vi "Constants.vi"() -> (14 "MetersInPixel":dbl, 15 "RobotLength(Px)":i16, 16 "RobotWidth(Px)":i16, 17 "PictureCenterPoint":cluster{"x":i16, "y":i16}={"x"=250, "y"=250})   [LabVIEW 2009, in "Host.lvlib" / "Draw.lvlib"]
uses:
  Draw.lvlib
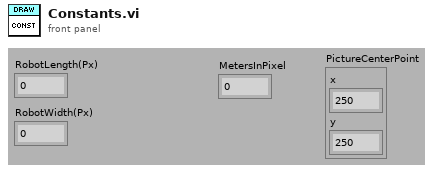
[diagram p1: front panel]
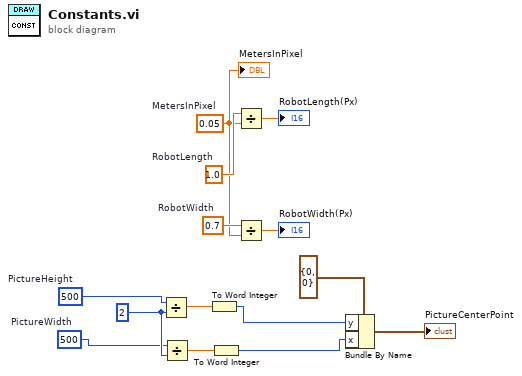
[diagram p0: block diagram]
diagram:
  w8 = i16 2 ("y")
  w7 = i16 500  # PictureWidth
  w9 = i16 500  # PictureHeight
  w12 = 0.7  # RobotWidth
  w14 = 1.0  # RobotLength
  w11 = 0.05  # MetersInPixel
  n1 = Divide(x=w9, y=w8) -> (x/y=w6:dbl)
  n2 = Divide(x=w7, y=w8) -> (x/y=w5:dbl)
  n3 = To Word Integer(number=w6) -> (16bit integer=w2:i16)
  n4 = To Word Integer(number=w5) -> (16bit integer=w1:i16)
  n5 = Divide(x=w14, y=w11) -> (x/y=→"RobotLength(Px)":dbl)
  n6 = Divide(x=w12, y=w11) -> (x/y=→"RobotWidth(Px)":dbl)
  n7 = Bundle By Name(cluster=cluster{"x":i16, "y":i16} {"x"=0, "y"=0} ("PictureCenterPoint 2"), "y"=w2, "x"=w1) -> (→"PictureCenterPoint":cluster{"x":i16, "y":i16})
  "MetersInPixel" <- w11
